vi "Get Status.vi"(8 "error in (no error)":errorcluster, 11 "FW Arduino Control in":refnum<class "FW Arduino Control.lvclass">) -> (0 "error out":errorcluster, 2 "FW Status":T1={"State"=enum."Move Complete", "Positions"=[], "Names"=[], "Notch"=[], "Moving"=[FALSE, FALSE]}, 3 "FW Arduino Control out":refnum<class "FW Arduino Control.lvclass">)   [LabVIEW 2024, in "FW Arduino Control.lvclass"]
uses:
  FW Arduino Control.lvclass
  FW cluster Status.ctl
  FW enum status.ctl
  Filter Wheel Object/Filter Wheel.lvclass
panel:
  out "reponses":string[](array[string])
  out "Moving":bool[](array[boolean])
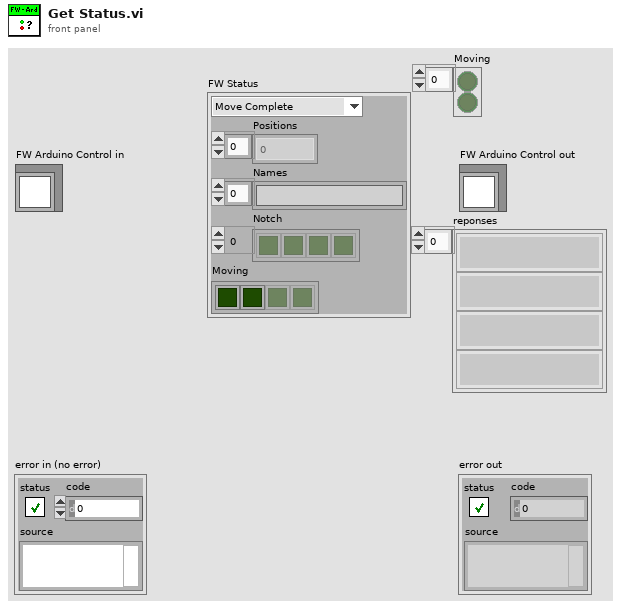
[diagram p1: front panel]
types:
  T1 = typedef "FW cluster Status.ctl" = cluster{"State":T2, "Positions":i32[], "Names":string[], "Notch":bool[], "Moving":bool[]}
  T2 = typedef "FW enum status.ctl" = enum16{"Initializing", "Moving", "Move Complete", "Error"}
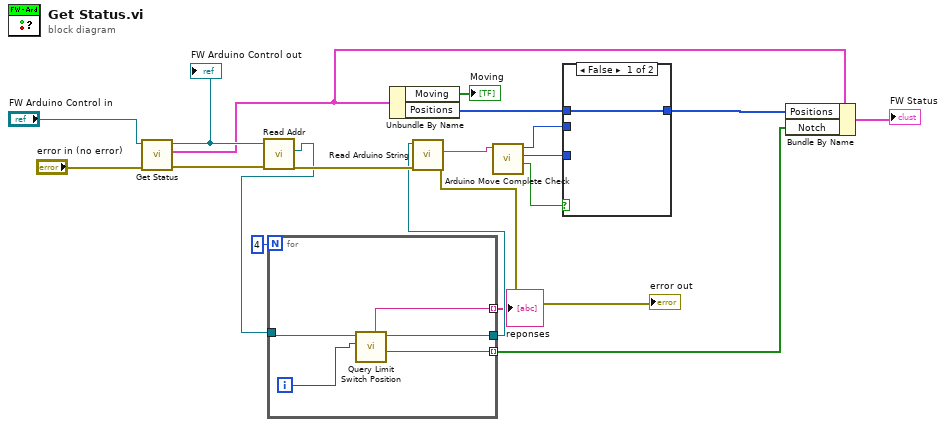
[diagram p0: block diagram]
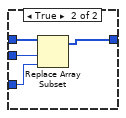
[diagram p2: hidden frame]
diagram:
  n1 = call-parent "Get Status.vi"("error in (no error)"="error in (no error)", "Filter Wheel in"="FW Arduino Control in") -> ("error out"=w14:errorcluster, "FW Status"=w2:T1, "Filter Wheel out"=w18:refnum<class "FW Arduino Control.lvclass">)  [unwired: 7 in]
  "FW Arduino Control out" <- w18
  n2 = call-dynamic "Read Addr.vi"("error in (no error)"=w14, "Filter Wheel in"=w18) -> ("error out"=w13:errorcluster, "Addr"=w7:refnum<visa-resource-name>)  [unwired: 7 in, 1 out]
  n3 = for {
    N: 4 -> [_]
    tunnel: w7 -> [w22]
    tunnel: [w25] -> w6
    tunnel: [w23] -> w5 mode=indexing
    tunnel: [w21] -> w1 mode=indexing
    i -> [w24]
    n4 = call "Query Limit Switch Position.vi"("motor (0:n-1)"=w24, "VISA resource name"=w22) -> ("At Switch?"=w23:bool, "reference out"=w25:refnum<visa-resource-name>, "response"=w21:string)  [unwired: 5 in, 2 out]
  }
  "reponses" <- w1
  n5 = Unbundle By Name(w2) -> ("Moving"=→"Moving":bool[], "Positions"=w17:i32[])
  n6 = call "Read Arduino String.vi"("error in (no error)"=w13, "reference"=w6) -> ("error out"=→"error out":errorcluster, "response"=w12:string)  [unwired: 7 in, 1 out]
  n7 = call "Arduino Move Complete Check.vi"("input string"=w12) -> ("Complete?"=w4:bool, "position"=w15:i32, "m"=w16:i32)  [unwired: 7 in, 1 out]
  n8 = case shown="False" w4 {
    tunnel: w17 -> [w26 w30]
    tunnel: w16 -> [_ w29]
    tunnel: w15 -> [_ w28]
    tunnel: [w26 w27] -> w10
    frame False {
    }
    frame True {
      n9 = Replace Array Subset(array=w30, new element=w28, index=w29) -> (w27:i32[])
    }
  }
  n10 = Bundle By Name(cluster=w2, "Positions"=w10, "Notch"=w5) -> (→"FW Status":T1)
